vi "Close.vi"(8 "Error In (no error)":errorcluster, 11 "VISA Resource Name":refnum<visa-resource-name>) -> (0 "Error Out":errorcluster)   [LabVIEW 2018, in "Agilent PNA Series.lvlib"]
doc: "This VI closes the I/O interface with the instrument."
uses:
  Agilent PNA Series.lvlib
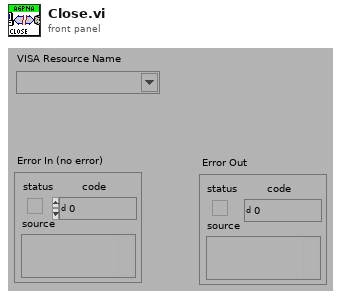
[diagram p1: front panel]
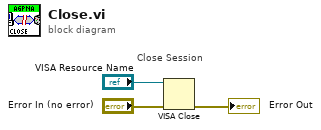
[diagram p0: block diagram]
diagram:
  # "Close Session"
  n1 = VISA Close(VISA resource name="VISA Resource Name", error in (no error)="Error In (no error)") -> (error out=→"Error Out":errorcluster)
